vi "AddEventDetect.vi"(5 "Edge":enum16{"Rising", "Falling", "Both"}(ring), 6 "Bounce time (msec)":i32, 7 "Channel":i32, 8 "error in":errorcluster) -> (0 "error out":errorcluster, 3 "Channel out":i32)   [LabVIEW 2014, in "GPIO.lvlib"]
doc: "Adds a value change event for the specified channel. Only one edge detection event is allowed per channel, if you need to change the edge type you must remove the existing event first.\n\nThe channel must be configured as an input before calling this VI."
uses:
  GPIO.lvlib
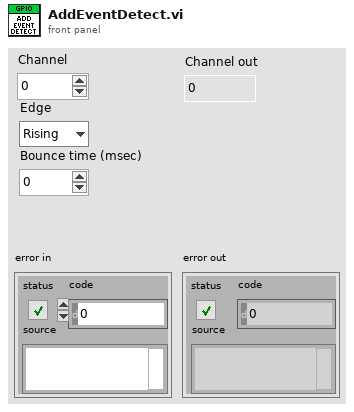
[diagram p1: front panel]
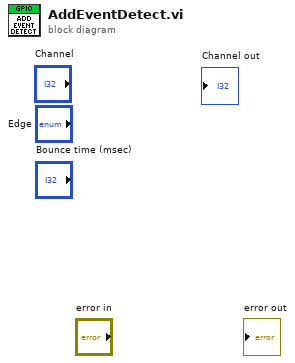
[diagram p0: block diagram]
diagram:
